vi "SysInfo-Expt VIs Version.vi"() -> (1 "Expt VIs Version out":i32)   [LabVIEW 2020]
panel:
  in  "Expt VIs Version":i32=2507
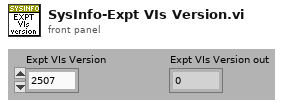
[diagram p1: front panel]
types:
  T1 = cluster{"Major":i32, "Minor":i32, "Build":i32, "Private":i32, "FileVersion":string, "ProductName":string, "InternalName":string, "CompanyName":string, "LegalCopyright":string, "FileDescription":string}
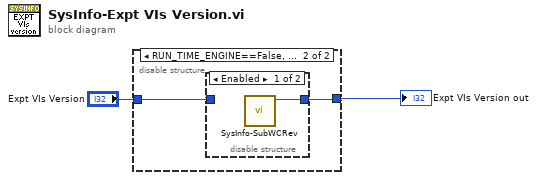
[diagram p0: block diagram]
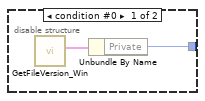
[diagram p2: hidden frame]
diagram:
  n1 = disable-structure shown="RUN_TIME_ENGINE==False, Default" {
    disable-tunnel: [w3 w6] -> w1
    disable-tunnel: "Expt VIs Version" -> [_ w5]
    frame condition #0 {
      n2 = call "GetFileVersion_Win.vi"() -> ("File Info Out"=w4:T1)  [unwired: 9 in, 2 out]
      n3 = Unbundle By Name(w4) -> ("Private"=w3:i32)
    }
    frame condition #1 (active) {
      n4 = disable-structure shown="Enabled" {
        disable-tunnel: [w7 w8] -> w6
        disable-tunnel: w5 -> [_ w8]
        frame Enabled {
          n5 = call "SysInfo-SubWCRev.vi"() -> ("Revision"=w7:i32)  [unwired: 9 in, 2 out]
        }
        frame Disabled {
        }
      }
    }
  }
  "Expt VIs Version out" <- w1
